vi "Algorithms.vi"() -> ()   [LabVIEW 2013]
uses:
  qwtb_lvlib/TD Algorithm Information.ctl
  globals.vi
panel:
  in  "curAlg":u16(ring) caption="Selected Algorithm ID" items=["INL", "PSFE", "testG", "testGM", "testM"]
  out "Algorithm Information":T1
  in  "reload alginfo":bool
  in  "close":bool
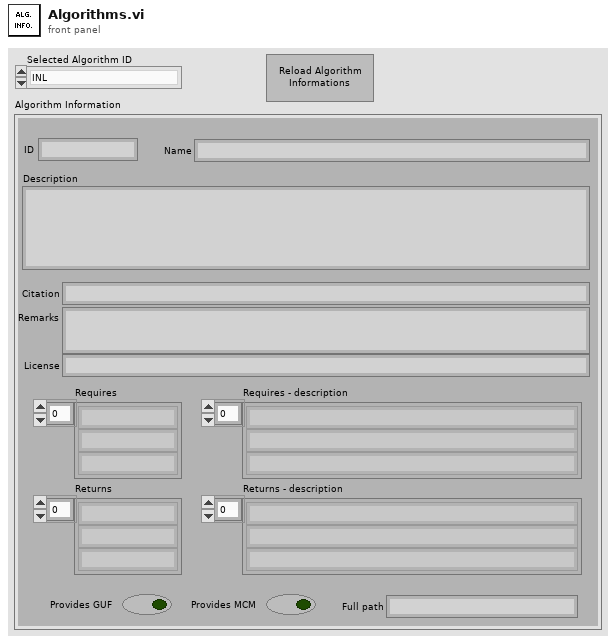
[diagram p1: front panel]
types:
  T1 = typedef "TD Algorithm Information.ctl" = cluster{"ID":string, "Name":string, "Description":string, "Citation":string, "Remarks":string, "License":string, "Requires":string[], "Requires - description":string[], "Returns":string[], "Returns - description":string[], "Provides GUF":bool, "Provides MCM":bool, "Full path":string}
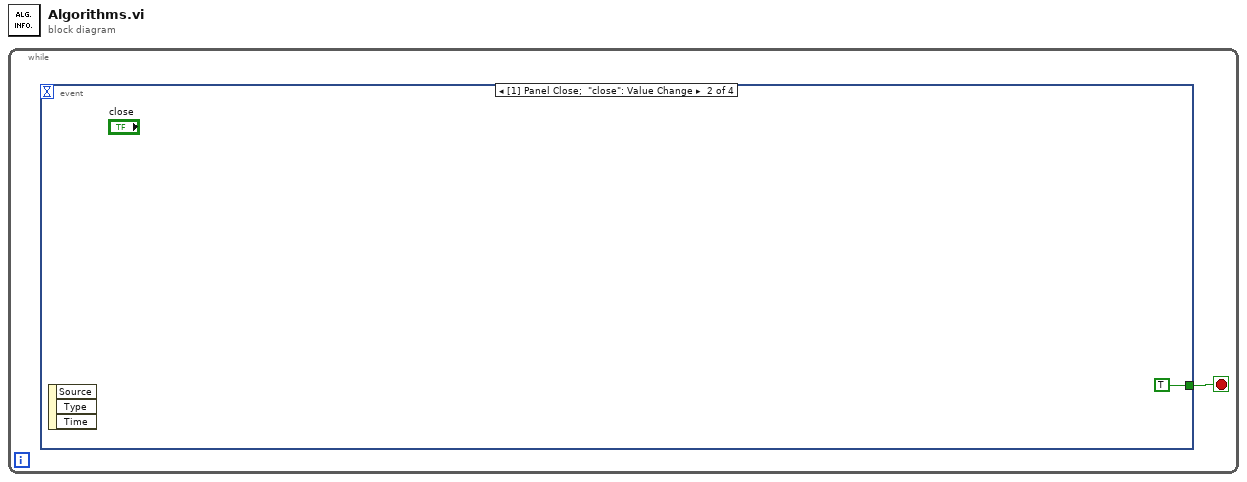
[diagram p0: block diagram]
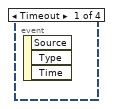
[diagram p2: hidden frame]
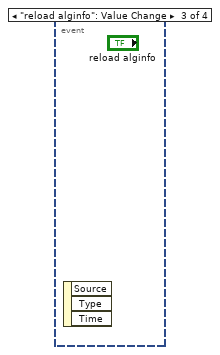
[diagram p3: hidden frame]
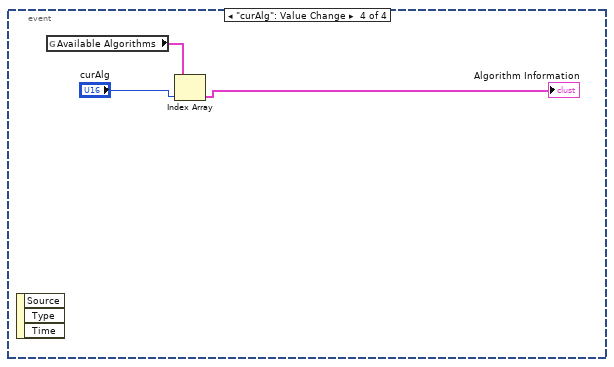
[diagram p4: hidden frame]
diagram:
  n1 = while {
    stop <- w1 stop-if-true
    n2 = event shown="[1] Panel Close;  \"close\": Value Change" {
      selector: _ -> [_ _ _ _]
      dyn-events: _ -> [_ _ _ _]
      timeout: _ -> [_ _ _ _]
      tunnel: [_ TRUE ("cancel") _ _] -> w1
      event Timeout {
        n3 = event-data() -> ()  [unwired: 1 in, 3 out]
      }
      event Panel Close; "close": Value Change {
        n4 = event-data() -> ()  [unwired: 1 in, 3 out]
      }
      event "reload alginfo": Value Change {
        n5 = event-data() -> ()  [unwired: 1 in, 3 out]
      }
      event "curAlg": Value Change {
        n6 = event-data() -> ()  [unwired: 1 in, 3 out]
        n7 = global read "globals.vi" "Available Algorithms"() -> (w5:T1[])
        n8 = Index Array(array=w5, index="curAlg") -> (element=→"Algorithm Information":T1)
      }
    }
  }
